vi "protoWindow_1.1.vi"() -> ()   [LabVIEW 2014]
uses:
  common/crest/LabVIEW/LV14/libcommon-crest.lvlib
panel:
  in  "Dataset":path=path "/home/chaos/chaos_bundle/driver/powersupply/Labview/LV14/crest/datasets/btf_20150320_1052.dat"
  out "keys out":string
  out "values out":string
  out "parameters":string
  out "command":string
  out "element":string
  in  "Current Set [A]":dbl format="%.3g"
  in  "set":bool
  in  "reset":bool
  in  "polaOpen":bool
  in  "polaPos":bool
  in  "polaNeg":bool
  out "fetch loop":i32
  out "index":i32
  in  "standby":bool
  in  "operational":bool
  in  "elementList":i32(listbox)
  in  "!CHAOS WAN url":string="192.168.150.91:8081"
  in  "enable window menu":bool
  in  "refreshConn":bool
  in  "set_to_saved":bool
  in  "local_load":bool
  in  "local_save":bool
  out "debug counter":i32
  # "ver. 1.1, build 20150320-1150"
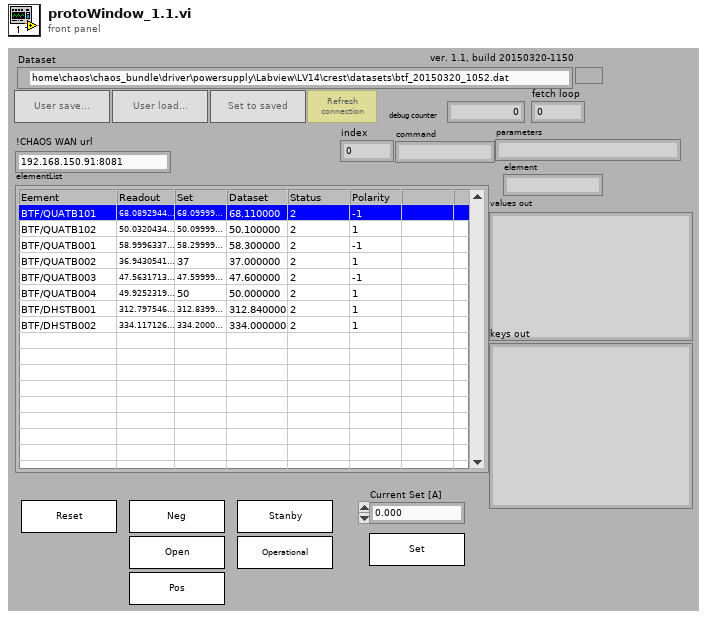
[diagram p1: front panel]
types:
  T1 = cluster{"numberOfElements":i32, "connectionHandle":u32, "selectedElement":i32}
  T2 = cluster{"currentReadout":string[], "currentSet":string[], "statusReadout":string[], "dataset":string[], "polarity":string[]}
  T3 = typedef "LVRectTypeDef.ctl" = cluster{"Left":i16, "Top":i16, "Right":i16, "Bottom":i16}
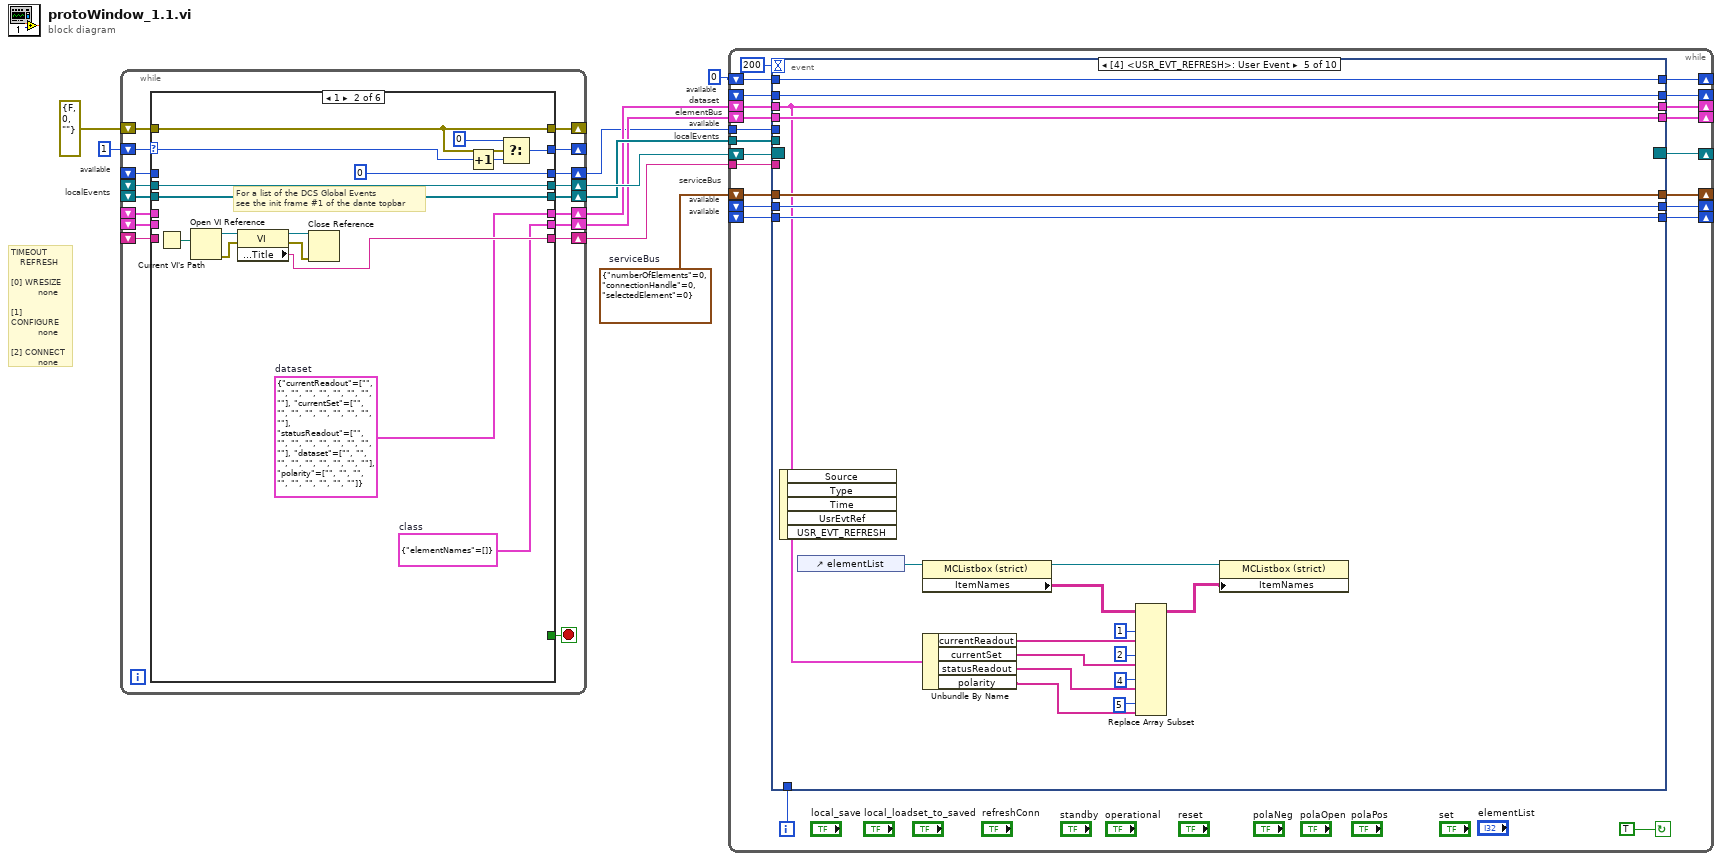
[diagram p0: block diagram]
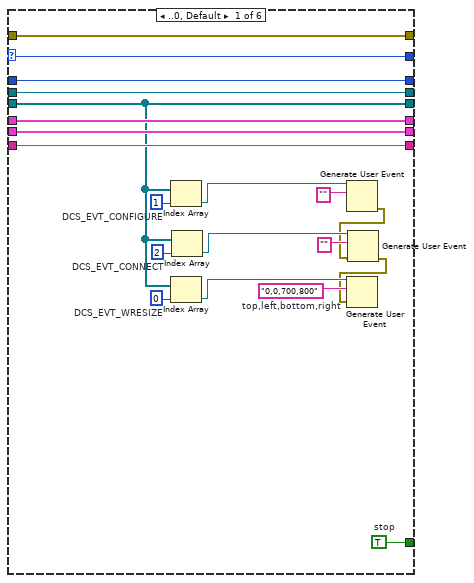
[diagram p2: hidden frame]
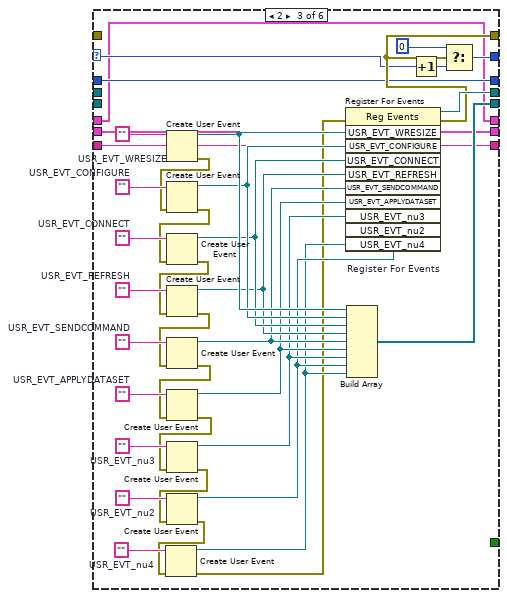
[diagram p3: hidden frame]
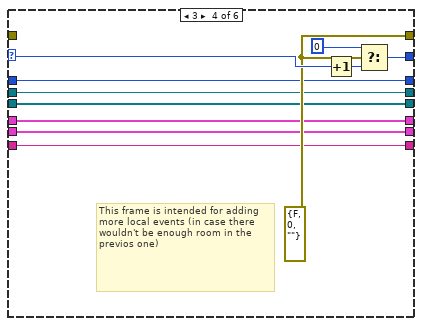
[diagram p4: hidden frame]
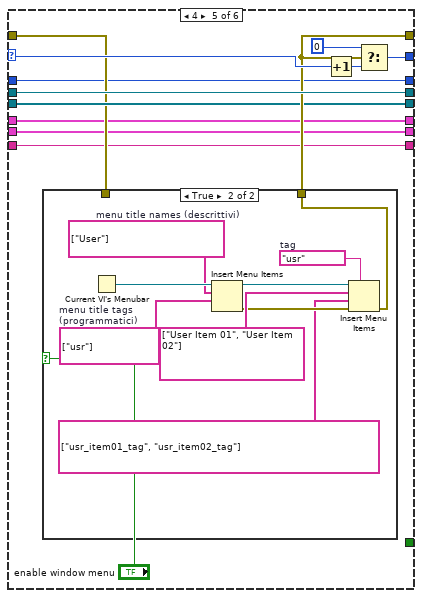
[diagram p5: hidden frame]
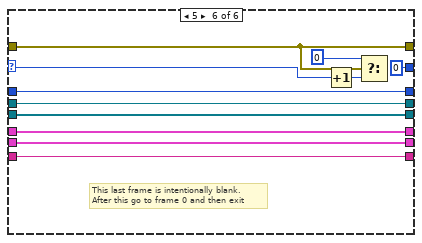
[diagram p7: hidden frame]
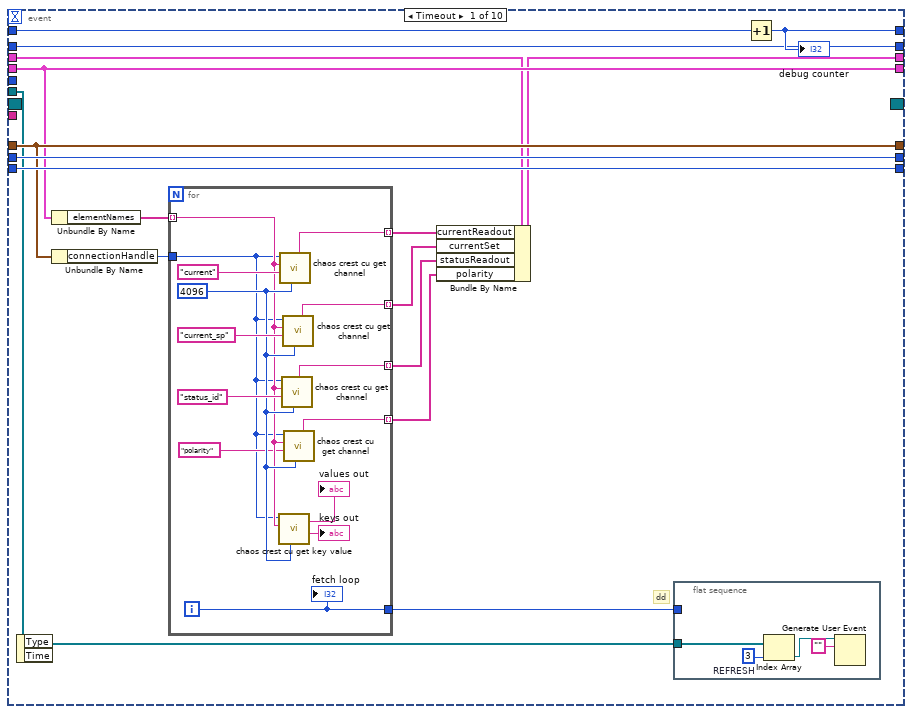
[diagram p8: hidden frame]
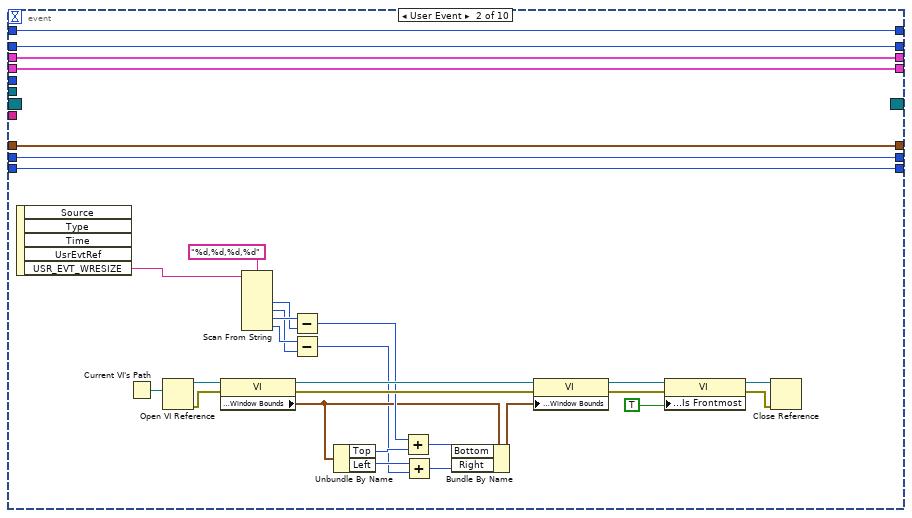
[diagram p9: hidden frame]
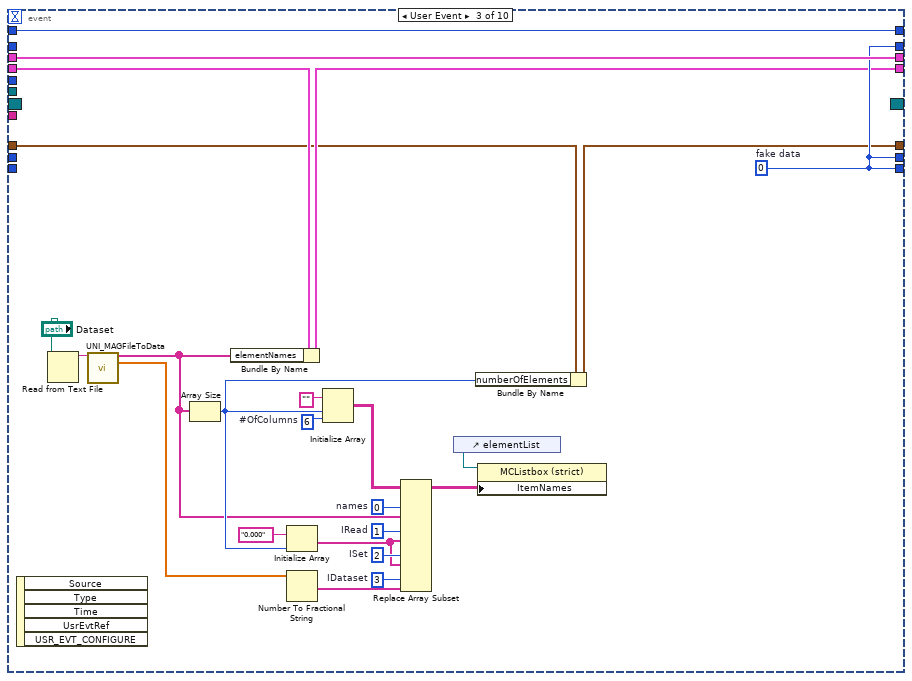
[diagram p10: hidden frame]
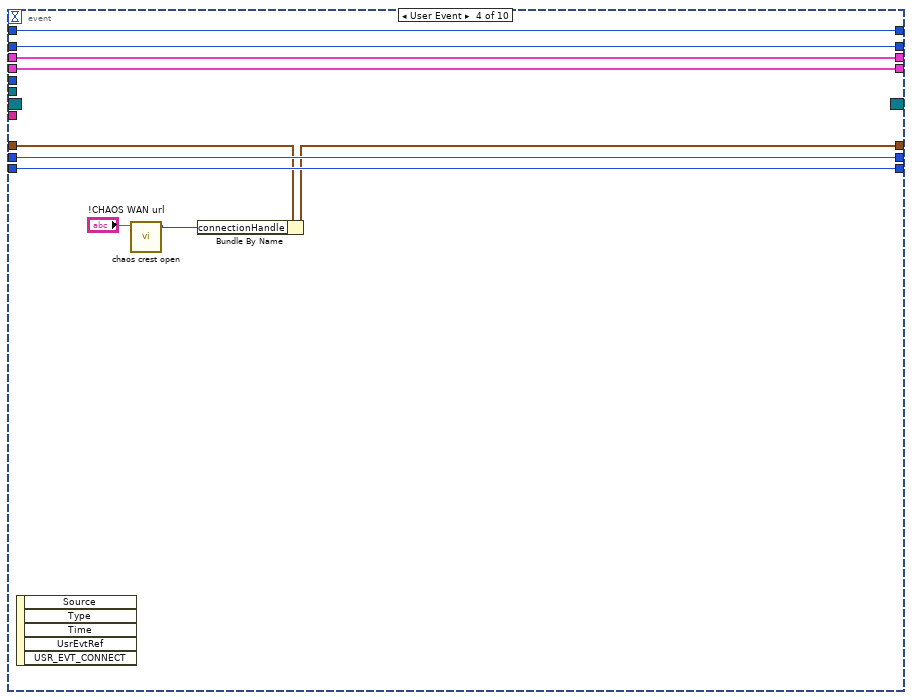
[diagram p11: hidden frame]
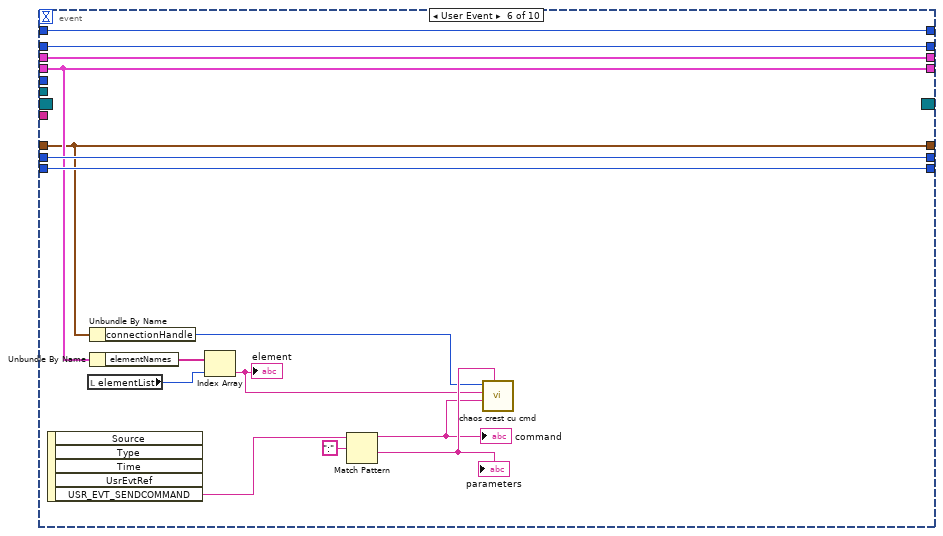
[diagram p12: hidden frame]
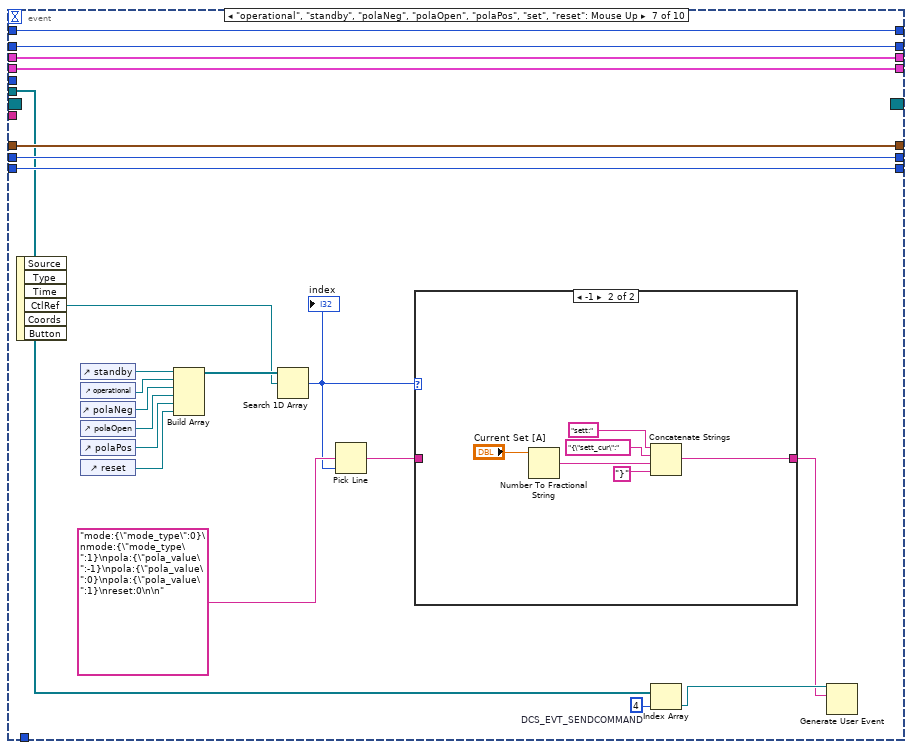
[diagram p13: hidden frame]
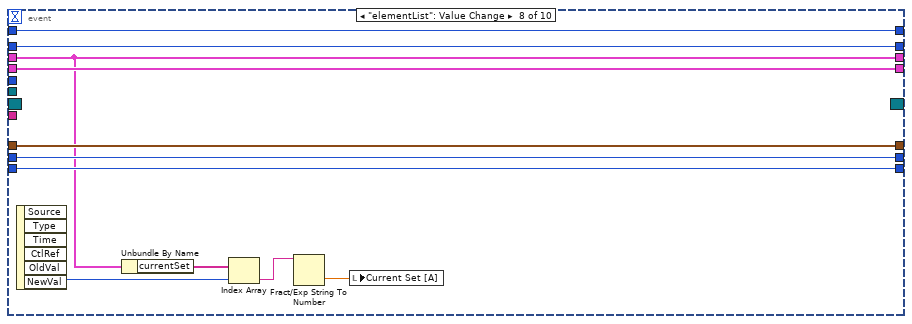
[diagram p15: hidden frame]
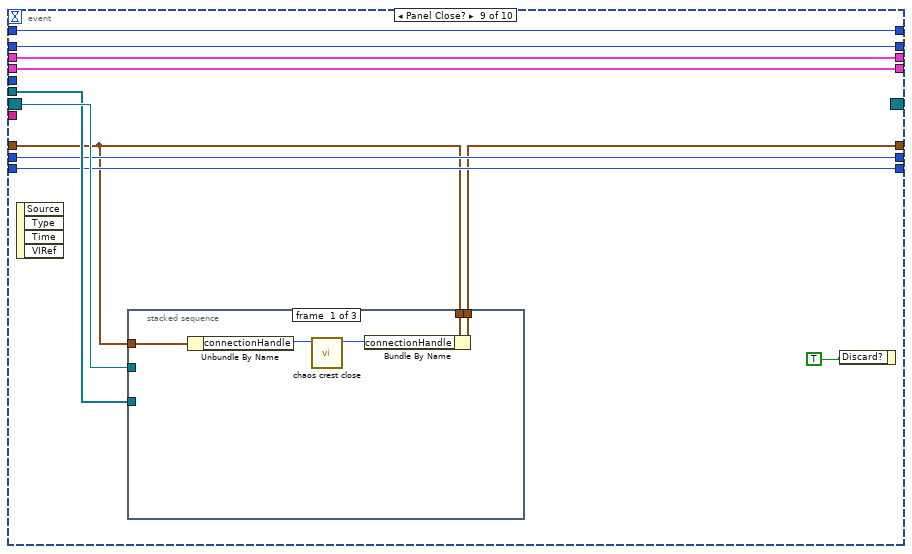
[diagram p16: hidden frame]
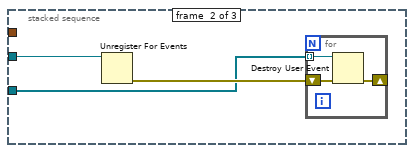
[diagram p17: hidden frame]
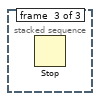
[diagram p18: hidden frame]
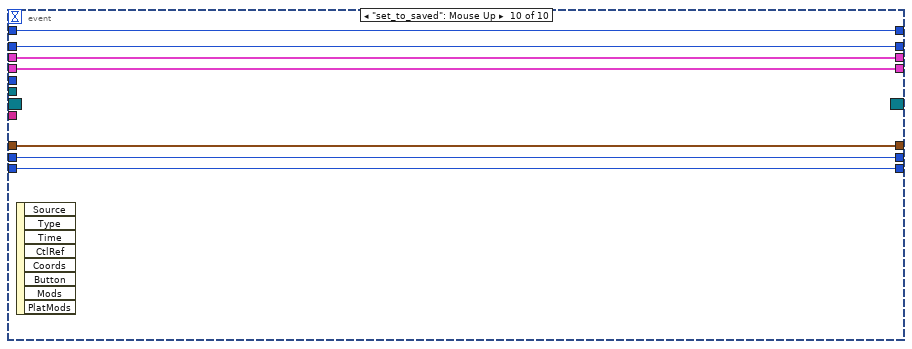
[diagram p19: hidden frame]
diagram:
  w4 = T1 {"numberOfElements"=0, "connectionHandle"=0, "selectedElement"=0}  # serviceBus
  # "available"
  # "serviceBus"
  # "TIMEOUT\n   REFRESH\n\n[0] WRESIZE\n         none\n\n[1] CONFIGURE\n         none\n\n[2] CONNECT\n         none"
  # "localEvents"
  # "available"
  # "localEvents"
  # "available"
  # "dataset"
  # "elementBus"
  # "available"
  # "available"
  n1 = while {
    shift-right: [w21] -> _
    shift-left: 1 -> [w24]
    shift-right: [w26] -> w8
    shift-left: _ -> [w23]
    shift-right: [w27] -> w6
    shift-left: _ -> [w22]
    shift-right: [w20] -> _
    shift-left: errorcluster {"status"=FALSE, "code"=0, "source"=""} ("error out") -> [w19]
    shift-right: [w18] -> w7
    shift-left: _ -> [w17]
    shift-right: [w16] -> w5
    shift-left: _ -> [w15]
    shift-right: [w14] -> w3
    shift-left: _ -> [w13]
    shift-right: [w12] -> w2
    shift-left: _ -> [w11]
    stop <- w25 stop-if-true
    n2 = case shown="1" w24 {
      tunnel: [w45 w49 w65 w104 w116 w140] -> w27
      tunnel: [w46 w63 w97 w106 w125 w143] -> w26
      selector: w24 -> [w43 w51 w92 w109 w121 w144]
      tunnel: [w47 _ _ _ _ _] -> w25
      tunnel: w23 -> [w46 w63 _ w106 w125 w143]
      tunnel: w22 -> [w45 _ w65 w104 w116 w140]
      tunnel: [w43 w53 w94 w110 w124 0 ("t")] -> w21
      tunnel: [w44 w52 w93 w108 w120 w137] -> w20
      tunnel: w19 -> [w44 w52 _ _ w117 w137]
      tunnel: [w28 w62 w91 w105 w119 w142] -> w18
      tunnel: w17 -> [w28 w62 _ w105 w119 w142]
      tunnel: [w42 w48 w64 w103 w115 w139] -> w16
      tunnel: w15 -> [w42 _ w64 w103 w115 w139]
      tunnel: [w38 0 w74 w107 w114 w138] -> w14
      tunnel: w13 -> [w38 _ w74 w107 w114 w138]
      tunnel: [w33 w56 w66 w102 w113 w136] -> w12
      tunnel: w11 -> [w33 _ w66 w102 w113 w136]
      frame ..0, Default {
        w32 = 1  # DCS_EVT_CONFIGURE
        w35 = 2  # DCS_EVT_CONNECT
        w39 = "0,0,700,800"  # top,left,bottom,right
        w41 = 0  # DCS_EVT_WRESIZE
        w47 = TRUE  # stop
        n3 = Index Array(array=w28, index=w32) -> (element=w31:refnum<user-event>)
        n4 = Index Array(array=w28, index=w41) -> (element=w40:refnum<user-event>)
        n5 = Index Array(array=w28, index=w35) -> (element=w36:refnum<user-event>)
        n6 = Generate User Event(user event=w31, event data cluster="" ("event data")) -> (error out=w29:errorcluster)  [unwired: 2 in, 1 out]
        n7 = Generate User Event(user event=w36, event data cluster="" ("event data"), error in=w29) -> (error out=w34:errorcluster)  [unwired: 1 in, 1 out]
        n8 = Generate User Event(user event=w40, event data cluster=w39, error in=w34) -> ()  [unwired: 1 in, 2 out]
      }
      frame 1 {
        w49 = T2 {"currentReadout"=["", "", "", "", "", "", "", "", ""], "currentSet"=["", "", "", "", "", "", "", "", ""], "statusReadout"=["", "", "", "", "", "", "", "", ""], "dataset"=["", "", "", "", "", "", "", "", ""], "polarity"=["", "", "", "", "", "", "", "", ""]}  # dataset
        w48 = cluster{"elementNames":string[]} {"elementNames"=[]}  # class
        # "For a list of the DCS Global Events\nsee the init frame #1 of the dante topbar"
        n9 = Current VI's Path() -> (path=w57:path)
        n10 = Open VI Reference(vi path=w57) -> (vi reference=w60:refnum<vi>, error out=w58:errorcluster)  [unwired: 5 in]
        n11 = property class="VI"(reference=w60, error in=w58) -> (reference out=w61:refnum<vi>, error out=w59:errorcluster, "Front Panel Window:Title"=w56:string)
        n12 = Close Reference(reference=w61, error in (no error)=w59) -> ()  [unwired: 1 out]
        n13 = Increment(x=w51) -> (x+1=w55:i32)
        n14 = Select(t=0, s=w52, f=w55) -> (s? t:f=w53:i32)
      }
      frame 2 {
        w70 = ""  # USR_EVT_nu4
        w73 = ""  # USR_EVT_nu2
        w80 = ""  # USR_EVT_nu3
        w83 = ""  # USR_EVT_APPLYDATASET
        w86 = ""  # USR_EVT_SENDCOMMAND
        w88 = ""  # USR_EVT_REFRESH
        w90 = ""  # USR_EVT_CONNECT
        w98 = ""  # USR_EVT_CONFIGURE
        w101 = ""  # USR_EVT_WRESIZE
        n15 = Create User Event(user event datatype=w101) -> (user event=w100:refnum<user-event>, error out=w77:errorcluster)  [unwired: 1 in]
        n16 = Create User Event(user event datatype=w98, error in=w77) -> (user event=w99:refnum<user-event>, error out=w76:errorcluster)
        n17 = Create User Event(user event datatype=w90, error in=w76) -> (user event=w89:refnum<user-event>, error out=w75:errorcluster)
        n18 = Create User Event(user event datatype=w88, error in=w75) -> (user event=w87:refnum<user-event>, error out=w85:errorcluster)
        n19 = Create User Event(user event datatype=w86, error in=w85) -> (user event=w84:refnum<user-event>, error out=w82:errorcluster)
        n20 = Create User Event(user event datatype=w83, error in=w82) -> (user event=w81:refnum<user-event>, error out=w79:errorcluster)
        n21 = Create User Event(user event datatype=w80, error in=w79) -> (user event=w78:refnum<user-event>, error out=w72:errorcluster)
        n22 = Create User Event(user event datatype=w73, error in=w72) -> (user event=w71:refnum<user-event>, error out=w69:errorcluster)
        n23 = Create User Event(user event datatype=w70, error in=w69) -> (user event=w68:refnum<user-event>, error out=w67:errorcluster)
        n24 = register-events "Register For Events"(error in=w67, w100, w99, w89, w87, w84, w81, w78, w71, w68) -> (reference out=w97:refnum<event-registration>, error out=w93:errorcluster)  [unwired: 1 in]
        n25 = Build Array(w100, w99, w89, w87, w84, w81, w78, w71, w68) -> (w91:refnum<user-event>[])
        n26 = Increment(x=w92) -> (x+1=w96:i32)
        n27 = Select(t=0, s=w93, f=w96) -> (s? t:f=w94:i32)
      }
      frame 3 {
        w108 = errorcluster {"status"=FALSE, "code"=0, "source"=""} ("s")
        # "This frame is intended for adding more local events (in case there wouldn't be enough room in the previos one)"
        n28 = Increment(x=w109) -> (x+1=w112:i32)
        n29 = Select(t=0, s=w108, f=w112) -> (s? t:f=w110:i32)
      }
      frame 4 {
        n30 = case shown="True" "enable window menu" {
          tunnel: [w126 w127] -> w120
          tunnel: w117 -> [w126 _]
          frame False {
          }
          frame True {
            w134 = string[] ["User"]  # menu title names (descrittivi)
            w132 = "usr"  # tag
            w129 = string[] ["usr"]  # menu title tags (programmatici)
            n31 = Current VI's Menubar() -> (w135:refnum<k9>)
            n32 = Insert Menu Items(7:w129, 8:w134, 9:w135) -> (0:w130:errorcluster, 3:w131:refnum<k9>)  [unwired: 3 in, 1 out]
            n33 = Insert Menu Items(5:w132, 6:w130, 7:string[] ["usr_item01_tag", "usr_item02_tag"] ("item names"), 8:string[] ["User Item 01", "User Item 02"] ("item names"), 9:w131) -> (0:w127:errorcluster)  [unwired: 1 in, 2 out]
          }
        }
        n34 = Increment(x=w121) -> (x+1=w123:i32)
        n35 = Select(t=0, s=w120, f=w123) -> (s? t:f=w124:i32)
      }
      frame 5 {
        # "This last frame is intentionally blank.\nAfter this go to frame 0 and then exit"
        n36 = Increment(x=w144) -> (x+1=w146:i32)
        n37 = Select(t=0, s=w137, f=w146) -> ()  [unwired: 1 out]
      }
    }
  }
  n38 = while {
    shift-right: [w153] -> _
    shift-left: w6 -> [w154]
    shift-right: [w155] -> _
    shift-left: w5 -> [w156]
    shift-right: [w165] -> _
    shift-left: _ -> [w166]
    shift-right: [w167] -> _
    shift-left: _ -> [w164]
    shift-right: [w161] -> _
    shift-left: w8 -> [w163]
    tunnel: w7 -> [w162]
    shift-right: [w158] -> _
    shift-left: w4 -> [w159]
    tunnel: w3 -> [w157]
    tunnel: w2 -> [w152]
    shift-right: [w150] -> _
    shift-left: 0 ("debug counter") -> [w151]
    shift-right: [w148] -> _
    shift-left: _ -> [w149]
    i -> [w147]
    stop <- TRUE continue-if-true
    n39 = event shown="[4] <USR_EVT_REFRESH>: User Event" {
      selector: w163 -> [_ _ _ _ _ _ _ _ w352 _]
      dyn-events: [_ _ _ _ _ _ _ _ _ _] -> w161
      timeout: 200 -> [_ _ _ _ _ _ _ _ _ _]
      tunnel: [w181 w233 w256 w268 w286 w301 w323 w341 w349 w370] -> w167
      tunnel: w166 -> [w185 w234 _ w267 w287 w302 w324 w342 w350 w371]
      tunnel: [w185 w234 w256 w267 w287 w302 w324 w342 w350 w371] -> w165
      tunnel: w164 -> [w181 w233 _ w268 w286 w301 w323 w341 w349 w370]
      tunnel: w162 -> [w178 _ _ _ _ _ w307 _ w351 _]
      tunnel: w159 -> [w180 w228 w243 w261 w285 w290 w320 w340 w344 w365]
      tunnel: [w180 w228 w242 w260 w285 w290 w320 w340 w343 w365] -> w158
      tunnel: w157 -> [_ _ _ _ _ _ _ _ _ _]
      tunnel: w156 -> [w176 w231 w254 w262 w284 w297 w318 w335 w347 w368]
      tunnel: [w176 w231 w253 w262 w284 w297 w318 w335 w347 w368] -> w155
      tunnel: w154 -> [w174 w232 w258 w264 w276 w300 w322 w334 w348 w369]
      tunnel: [w173 w232 w258 w264 w276 w300 w322 w334 w348 w369] -> w153
      tunnel: w152 -> [_ _ _ _ _ _ _ _ _ _]
      tunnel: w151 -> [w184 w227 w257 w266 w283 w299 w321 w339 w346 w367]
      tunnel: [w183 w227 w257 w266 w283 w299 w321 w339 w346 w367] -> w150
      tunnel: [w182 w226 w256 w265 w282 w298 w319 w338 w345 w366] -> w148
      tunnel: w149 -> [w182 w226 _ w265 w282 w298 w319 w338 w345 w366]
      tunnel: w147 -> [_ _ _ _ _ _ _ _ _ _]
      event Timeout {
        # "dd"
        n40 = event-data() -> ()  [unwired: 1 in, 2 out]
        n41 = Unbundle By Name(w176) -> ("elementNames"=w175:string[])
        n42 = Unbundle By Name(w180) -> ("connectionHandle"=w179:u32)
        n43 = for {
          tunnel: w179 -> [w191]
          tunnel: [w202] -> w172 mode=indexing
          tunnel: [w201] -> w177
          tunnel: w175 -> [w193] mode=indexing
          tunnel: [w198] -> w171 mode=indexing
          tunnel: [w196] -> w170 mode=indexing
          tunnel: [w190] -> w169 mode=indexing
          i -> [w201]
          w194 = 4096 ("maxsize")
          n44 = call "chaos crest cu get key value.vi"("maxsize"=w194, "cuname"=w193, "handleConnection"=w191) -> ("keys out"=→"keys out":string, "values out"=→"values out":string)  [unwired: 5 in, 2 out]
          n45 = call "chaos crest cu get channel.vi"("maxsize"=w194, "channame"="current", "cuname"=w193, "handleConnection"=w191) -> ("value out"=w202:string)  [unwired: 6 in, 1 out]
          n46 = call "chaos crest cu get channel.vi"("maxsize"=w194, "channame"="status_id", "cuname"=w193, "handleConnection"=w191) -> ("value out"=w196:string)  [unwired: 6 in, 1 out]
          n47 = call "chaos crest cu get channel.vi"("maxsize"=w194, "channame"="current_sp", "cuname"=w193, "handleConnection"=w191) -> ("value out"=w198:string)  [unwired: 6 in, 1 out]
          n48 = call "chaos crest cu get channel.vi"("maxsize"=w194, "channame"="polarity", "cuname"=w193, "handleConnection"=w191) -> ("value out"=w190:string)  [unwired: 6 in, 1 out]
          "fetch loop" <- w201
        }
        n49 = Bundle By Name(cluster=w174, "currentReadout"=w172, "currentSet"=w171, "statusReadout"=w170, "polarity"=w169) -> (w173:T2)
        n50 = flat-sequence {
          tunnel: w178 -> [w186]
          tunnel: w177 -> [_]
          frame #0 {
            w187 = 3  # REFRESH
            n51 = Index Array(array=w186, index=w187) -> (element=w188:refnum<user-event>)
            n52 = Generate User Event(user event=w188, event data cluster="" ("event data")) -> ()  [unwired: 2 in, 2 out]
          }
        }
        n53 = Increment(x=w184) -> (x+1=w183:i32)
        "debug counter" <- w183
      }
      event User Event {
        n54 = event-data() -> ("USR_EVT_WRESIZE"=w229:string)  [unwired: 1 in, 4 out]
        n55 = Current VI's Path() -> (path=w220:path)
        n56 = Open VI Reference(vi path=w220) -> (vi reference=w219:refnum<vi>, error out=w218:errorcluster)  [unwired: 5 in]
        n57 = property class="VI"(reference=w219, error in=w218) -> (reference out=w216:refnum<vi>, error out=w217:errorcluster, "Front Panel Window:Window Bounds"=w212:T3)
        n58 = Scan From String(format string="%d,%d,%d,%d", input string=w229) -> (output 1=w214:i32, output 2=w207:i32, output 3=w215:i32, output 4=w208:i32)  [unwired: 6 in, 3 out]
        n59 = Subtract(x=w215, y=w214) -> (x-y=w213:i32)
        n60 = Subtract(x=w208, y=w207) -> (x-y=w205:i32)
        n61 = Unbundle By Name(w212) -> ("Top"=w210:i16, "Left"=w206:i16)
        n62 = Add(x=w213, y=w210) -> (x+y=w209:i32)
        n63 = Add(x=w206, y=w205) -> (x+y=w204:i32)
        n64 = Bundle By Name(cluster=w212, "Bottom"=w209, "Right"=w204) -> (w211:T3)
        n65 = property class="VI"(reference=w216, error in=w217, "Front Panel Window:Window Bounds"=w211) -> (reference out=w221:refnum<vi>, error out=w222:errorcluster)
        n66 = property class="VI"(reference=w221, error in=w222, "Front Panel Window:Is Frontmost"=TRUE) -> (reference out=w224:refnum<vi>, error out=w225:errorcluster)
        n67 = Close Reference(reference=w224, error in (no error)=w225) -> ()  [unwired: 1 out]
      }
      event User Event {
        w237 = 3  # IDataset
        w245 = 2  # ISet
        w247 = 1  # IRead
        w241 = 6  # #OfColumns
        w252 = 0  # names
        w256 = 0  # fake data
        n68 = event-data() -> ()  [unwired: 1 in, 5 out]
        n69 = Read from Text File(file (use dialog)="Dataset") -> (text=w255:string)  [unwired: 3 in, 3 out]
        n70 = call "UNI_MAGFileToData.vi"("spreadsheetData"=w255) -> ("names"=w239:string[], "settings"=w236:dbl[])  [unwired: 6 in, 7 out]
        n71 = Array Size(array=w239) -> (size(s)=w240:i32)
        n72 = Bundle By Name(cluster=w254, "elementNames"=w239) -> (w253:cluster{"elementNames":string[]})
        n73 = Initialize Array("0.000" ("event data"), w240) -> (w244:string[])
        n74 = Number To Fractional String(number=w236) -> (F-format string=w235:string[])  [unwired: 3 in]
        n75 = Initialize Array("" ("event data"), w240, w241) -> (w248:string[][])
        n76 = Replace Array Subset(array=w248, new element #1=w239, index (col) #1=w252, new element #2=w244, index (col) #2=w247, new element #3=w244, index (col) #3=w245, new element #4=w235, index (col) #4=w237) -> (w251:string[][])  [unwired: 4 in]
        n77 = control-ref of="elementList"() -> (w250:refnum<vi>)
        n78 = Bundle By Name(cluster=w243, "numberOfElements"=w240) -> (w242:T1)
        n79 = property class="MCListbox (strict)"(reference=w250, "ItemNames"=w251) -> ()  [unwired: 1 in, 2 out]
      }
      event User Event {
        n80 = event-data() -> ()  [unwired: 1 in, 5 out]
        n81 = call "chaos crest open.vi"("chaoswanurl"="!CHAOS WAN url") -> ("handleConnection"=w259:u32)  [unwired: 10 in]
        n82 = Bundle By Name(cluster=w261, "connectionHandle"=w259) -> (w260:T1)
      }
      event User Event {
        n83 = event-data() -> ()  [unwired: 1 in, 5 out]
        n84 = control-ref of="elementList"() -> (w280:refnum<vi>)
        n85 = property class="MCListbox (strict)"(reference=w280) -> (reference out=w279:refnum<vi>, "ItemNames"=w278:string[][])  [unwired: 1 in, 1 out]
        n86 = Unbundle By Name(w276) -> ("currentReadout"=w275:string[], "currentSet"=w273:string[], "statusReadout"=w271:string[], "polarity"=w269:string[])
        n87 = Replace Array Subset(array=w278, new element #1=w275, index (col) #1=1 ("disabled index (col)"), new element #2=w273, index (col) #2=2 ("disabled index (col)"), new element #3=w271, index (col) #3=4 ("disabled index (col)"), new element #4=w269, index (col) #4=5 ("disabled index (col)")) -> (w277:string[][])  [unwired: 4 in]
        n88 = property class="MCListbox (strict)"(reference=w279, "ItemNames"=w277) -> ()  [unwired: 1 in, 2 out]
      }
      event User Event {
        n89 = event-data() -> ("USR_EVT_SENDCOMMAND"=w293:string)  [unwired: 1 in, 4 out]
        n90 = local read "elementList"() -> (w295:i32)
        n91 = Unbundle By Name(w290) -> ("connectionHandle"=w289:u32)
        n92 = Unbundle By Name(w297) -> ("elementNames"=w296:string[])
        n93 = Index Array(array=w296, index=w295) -> (element=w288:string)
        "element" <- w288
        n94 = Match Pattern(string=w293, regular expression=":") -> (before substring=w291:string, after substring=w292:string)  [unwired: 1 in, 2 out]
        "command" <- w291
        "parameters" <- w292
        n95 = call "chaos crest cu cmd.vi"("args"=w292, "cmd"=w291, "cuname"=w288, "handleConnection"=w289) -> ()  [unwired: 7 in, 1 out]
      }
      event "operational", "standby", "polaNeg", "polaOpen", "polaPos", "set", "reset": Mouse Up {
        w309 = 4  # DCS_EVT_SENDCOMMAND
        n96 = event-data() -> ("CtlRef"=w316:refnum<vi>)  [unwired: 1 in, 5 out]
        n97 = control-ref of="standby"() -> (w314:refnum<vi>)
        n98 = control-ref of="operational"() -> (w313:refnum<vi>)
        n99 = control-ref of="polaNeg"() -> (w312:refnum<vi>)
        n100 = control-ref of="polaOpen"() -> (w311:refnum<vi>)
        n101 = control-ref of="polaPos"() -> (w310:refnum<vi>)
        n102 = control-ref of="reset"() -> (w303:refnum<vi>)
        n103 = Build Array(w314, w313, w312, w311, w310, w303) -> (w317:refnum<vi>[])
        n104 = Search 1D Array(1D array=w317, element=w316) -> (index of element=w304:i32)  [unwired: 1 in]
        "index" <- w304
        n105 = Pick Line(multi-line string="mode:{\"mode_type\":0}\nmode:{\"mode_type\":1}\npola:{\"pola_value\":-1}\npola:{\"pola_value\":0}\npola:{\"pola_value\":1}\nreset:0\n\n", line index=w304) -> (output string=w306:string)  [unwired: 1 in]
        n106 = case shown="-1" w304 {
          tunnel: w306 -> [w325 _]
          tunnel: [w325 w327] -> w305
          frame Default {
          }
          frame -1 {
            n107 = Number To Fractional String(number="Current Set [A]") -> (F-format string=w329:string)  [unwired: 3 in]
            n108 = Concatenate Strings("sett:" ("cmd"), "{\"sett_cur\":", w329, "}" ("string")) -> (w327:string)
          }
        }
        n109 = Index Array(array=w307, index=w309) -> (element=w308:refnum<user-event>)
        n110 = Generate User Event(user event=w308, event data cluster=w305) -> ()  [unwired: 2 in, 2 out]
      }
      event "elementList": Value Change {
        n111 = event-data() -> ("NewVal"=w336:i32)  [unwired: 1 in, 5 out]
        n112 = Unbundle By Name(w334) -> ("currentSet"=w337:string[])
        n113 = Index Array(array=w337, index=w336) -> (element=w333:string)
        n114 = Fract/Exp String To Number(string=w333) -> (number=w332:dbl)  [unwired: 3 in, 1 out]
        n115 = local write "Current Set [A]"(w332) -> ()
      }
      event Panel Close? {
        n116 = event-data() -> ()  [unwired: 1 in, 4 out]
        n117 = stacked-sequence {
          tunnel: w352 -> [_ w360 _]
          tunnel: w351 -> [_ w359 _]
          tunnel: w344 -> [w357 _ _]
          tunnel: w344 -> [w356 _ _]
          tunnel: [w355 _ _] -> w343
          frame #0 {
            n118 = Unbundle By Name(w357) -> ("connectionHandle"=w358:u32)
            n119 = call "chaos crest close.vi"("connectionHandle"=w358) -> ("connectionHandle out"=w354:u32)  [unwired: 9 in, 1 out]
            n120 = Bundle By Name(cluster=w356, "connectionHandle"=w354) -> (w355:T1)
          }
          frame #1 {
            n121 = Unregister For Events(event registration refnum=w360) -> (error out=w361:errorcluster)  [unwired: 1 in]
            n122 = for {
              tunnel: w359 -> [w364] mode=indexing
              shift-right: [w362] -> _
              shift-left: w361 -> [w363]
              n123 = Destroy User Event(user event=w364, error in=w363) -> (error out=w362:errorcluster)
            }
          }
          frame #2 {
            n124 = Stop() -> ()  [unwired: 1 in]
          }
        }
        n125 = event-data("Discard?"=TRUE) -> ()  [unwired: 1 in, 1 out]
      }
      event "set_to_saved": Mouse Up {
        n126 = event-data() -> ()  [unwired: 1 in, 8 out]
      }
    }
  }
